vi "LegendSettings(SubVI).vi"(8 "Error In":errorcluster, 9 "Legend":refnum<vi>, 10 "XYGraph Refnum":refnum<vi>, 11 "Arr Refnum":refnum<vi>) -> (0 "Error Out":errorcluster)   [LabVIEW 2018]
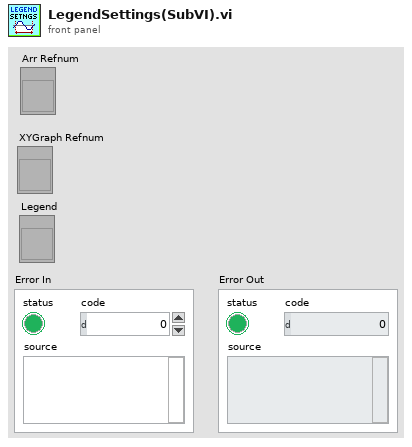
[diagram p1: front panel]
types:
  T1 = typedef "Line.ctl" = cluster{"Width":dbl, "Color":i64, "Array Oy":dbl[], "Array Ox":dbl[], "Name":string, "Plot Visible":T2}
  T2 = typedef "View.ctl" = bool
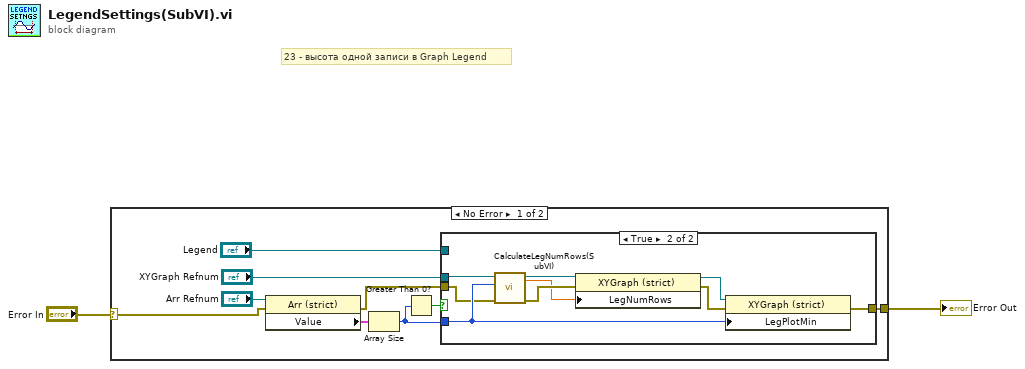
[diagram p0: block diagram]
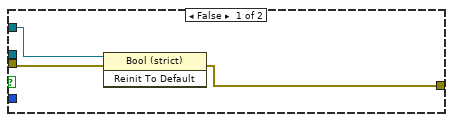
[diagram p2: hidden frame]
diagram:
  # "23 - высота одной записи в Graph Legend"
  n1 = case shown="No Error" "Error In" {
    selector: "Error In" -> [w6 w24]
    tunnel: [w4 w24] -> w1
    frame No Error {
      n2 = property on="Property Node" class="Arr (strict)"(reference="Arr Refnum", error in=w6) -> (error out=w5:errorcluster, "Value"=w7:T1[])  [unwired: 1 out]
      n3 = Array Size(array=w7) -> (size(s)=w11:i32)
      n4 = Greater Than 0?(x=w11) -> (x > 0?=w10:bool)
      n5 = case shown="True" w10 {
        tunnel: w11 -> [_ w19]
        tunnel: "XYGraph Refnum" -> [_ w20]
        tunnel: "Legend" -> [w14 _]
        tunnel: w5 -> [w13 w18]
        tunnel: [w12 w21] -> w4
        frame False {
          n6 = invoke on="Invoke Node" class="Bool (strict)" method="Reinit To Default"(reference=w14, error in=w13) -> (error out=w12:errorcluster)  [unwired: 1 in, 2 out]
        }
        frame True {
          n7 = call "CalculateLegNumRows(SubVI).vi"("Error In"=w18, "PlotsNum"=w19, "XYGraph in"=w20) -> ("Error Out"=w17:errorcluster, "LegNumRows"=w15:dbl, "XYGraph in 2"=w16:refnum<vi>)  [unwired: 6 in]
          n8 = property on="Property Node" class="XYGraph (strict)"(reference=w16, error in=w17, "LegNumRows"=w15) -> (reference out=w22:refnum<vi>, error out=w23:errorcluster)
          n9 = property on="Property Node" class="XYGraph (strict)"(reference=w22, error in=w23, "LegPlotMin"=w19) -> (error out=w21:errorcluster)  [unwired: 1 out]
        }
      }
    }
    frame Error {
    }
  }
  "Error Out" <- w1
